vi "FdxCmdTMControlCvi.vi"(8 "error in":errorcluster, 9 "TM_ControlIn":T1, 10 "TMHandle":u32, 11 "InstrumentHandle":u32) -> (0 "error out":errorcluster, 2 "TMHandleOut":u32, 3 "InstrumentHandle":u32)   [LabVIEW 2020, in "AIM664LV.lvlib"]
doc: "This function is used to start and stop a Time Manager. Note: the Tx and Rx Ports must be started prior to the Time Manager with calls to FdxCmdTxControl and FdxCmdRxControl in order to enable the Time Manager to send and receive data."
uses:
  AIM664LV.lvlib
  AFDX_LibraryAdmin/FdxGlobalDllPath.vi
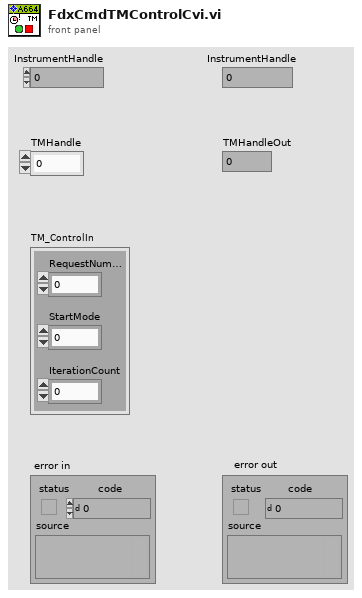
[diagram p1: front panel]
types:
  T1 = cluster{"RequestNumber":u16, "StartMode":u32, "IterationCount":u32}
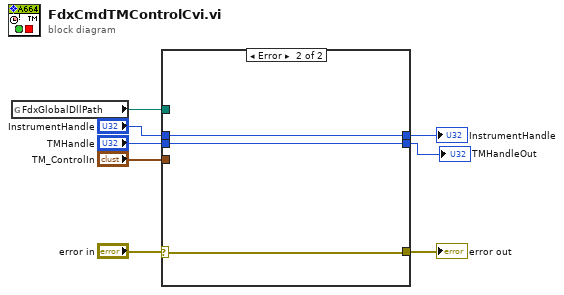
[diagram p0: block diagram]
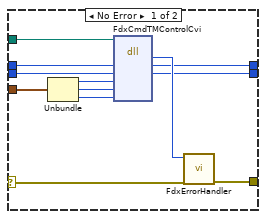
[diagram p2: hidden frame]
diagram:
  n1 = global read "FdxGlobalDllPath.vi" "FdxGlobalDllPath"() -> (w6:path)
  n2 = case shown="Error" "error in" {
    selector: "error in" -> [w19 w23]
    tunnel: [w20 w23] -> w8
    tunnel: w6 -> [w14 _]
    tunnel: "InstrumentHandle" -> [w13 w22]
    tunnel: [w12 w22] -> w4
    tunnel: "TM_ControlIn" -> [w11 _]
    tunnel: "TMHandle" -> [w10 w21]
    tunnel: [w9 w21] -> w1
    frame No Error {
      n3 = Unbundle(w11) -> ("RequestNumber"=w17:u16, "StartMode"=w16:u32, "IterationCount"=w15:u32)
      n4 = dll-call lib="aim_fdx.19.dll" fn="FdxCmdTMControlCvi"(path in=w14, "InstrumentHandle"=w13, "TMHandle"=w10, "RequestNumber"=w17, "StartMode"=w16, "IterationCount"=w15) -> ("status"=w18:i32, "InstrumentHandle"=w12:u32, "TMHandle"=w9:u32)  [unwired: 5 in, 2 out]
      n5 = call "FdxErrorHandler.vi"("error in"=w19, "AIM Error"=w18) -> ("error out"=w20:errorcluster)  [unwired: 9 in]
    }
    frame Error {
    }
  }
  "error out" <- w8
  "InstrumentHandle" <- w4
  "TMHandleOut" <- w1
